vi "Capture@Config__Parameter.vi"(1 "ParamterIn":string) -> (0 "ParamterOut":string)   [LabVIEW 2019]
panel:
  in  "Param":string(combo)
  in  "Config":string(combo)
  in  "CamName":string(combo)
  in  "Confirm":bool
  # "Capture@AddCAM $Capture,$Paramter,$Value"
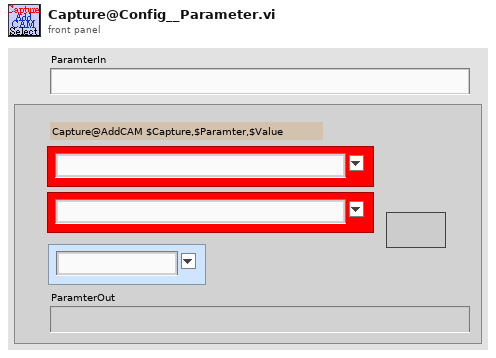
[diagram p1: front panel]
types:
  T1 = enum16{"AddCam", "GetIndex", "Init", "GetList", "SetInfo"}
  T2 = cluster{"Init?":bool, "DeviceName":string, "DeviceInfo":variant, "error state":errorcluster, "Stop":bool}
  T3 = cluster{"Init":refnum<vi>, "Close":refnum<vi>, "Config":refnum<vi>, "NOP":refnum<vi>, "Snapshot":refnum<vi>, "Trigger":refnum<vi>, "GetConfig":refnum<vi>}
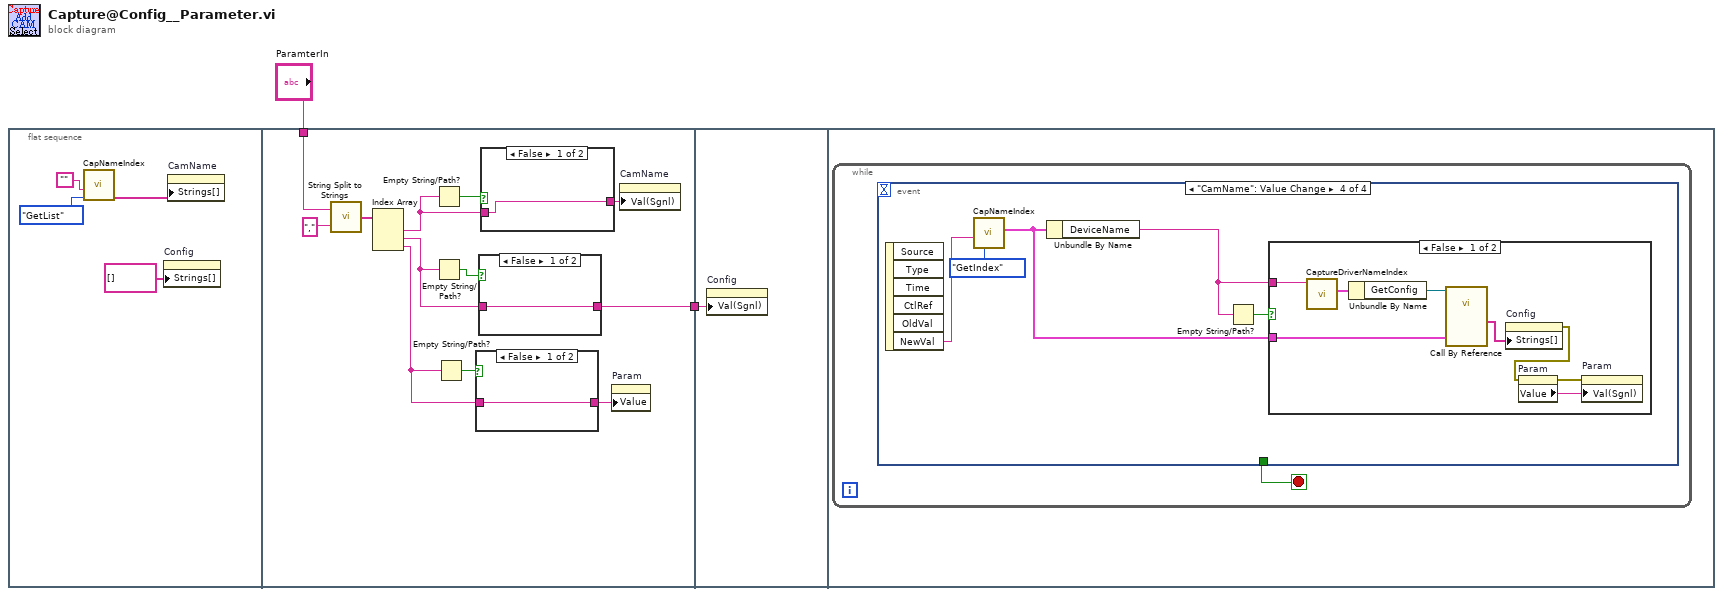
[diagram p0: block diagram]
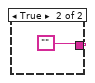
[diagram p2: hidden frame]
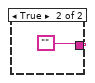
[diagram p3: hidden frame]
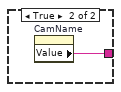
[diagram p4: hidden frame]
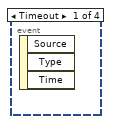
[diagram p5: hidden frame]
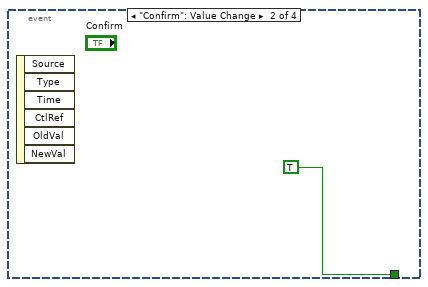
[diagram p6: hidden frame]
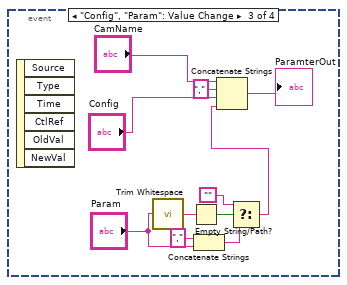
[diagram p7: hidden frame]
diagram:
  n1 = flat-sequence {
    tunnel: "ParamterIn" -> [w16]
    tunnel: [w8] -> w1
    tunnel: w1 -> [w25]
    frame #0 {
      n2 = call "CapNameIndex.vi"("OP"=enum16{"AddCam", "GetIndex", "Init", "GetList"}."GetList", "CamName"="") -> ("DeviceList"=w5:string[])  [unwired: 2 in, 3 out]
      n3 = property on="Config" class="CmbBox"("Strings[]"=string[] [] ("Strings []")) -> ()  [unwired: 2 in, 2 out]
      n4 = property on="CamName" class="CmbBox"("Strings[]"=w5) -> ()  [unwired: 2 in, 2 out]
    }
    frame #1 {
      n5 = call "String Split to Strings.vi"("search string/char (-)"=",", "String"=w16) -> ("Array"=w18:string[])
      n6 = Index Array(array=w18) -> (element #1=w14:string, element #2=w12:string, element #3=w10:string)  [unwired: 3 in]
      n7 = Empty String/Path?(string/path=w14) -> (empty?=w15:bool)
      n8 = Empty String/Path?(string/path=w12) -> (empty?=w13:bool)
      n9 = Empty String/Path?(string/path=w10) -> (empty?=w11:bool)
      n10 = case shown="False" w11 {
        tunnel: [w19 ""] -> w9
        tunnel: w10 -> [w19 _]
        frame False {
        }
        frame True {
        }
      }
      n11 = case shown="False" w13 {
        tunnel: [w21 ""] -> w8
        tunnel: w12 -> [w21 _]
        frame False {
        }
        frame True {
        }
      }
      n12 = case shown="False" w15 {
        tunnel: w14 -> [w23 _]
        tunnel: [w23 w24] -> w7
        frame False {
        }
        frame True {
          n13 = property on="CamName" class="CmbBox"() -> ("Value"=w24:string)  [unwired: 2 in, 2 out]
        }
      }
      n14 = property on="Param" class="CmbBox"("Value"=w9) -> ()  [unwired: 2 in, 2 out]
      n15 = property on="CamName" class="CmbBox"("Val(Sgnl)"=w7) -> ()  [unwired: 2 in, 2 out]
    }
    frame #2 {
      n16 = property on="Config" class="CmbBox"("Val(Sgnl)"=w25) -> ()  [unwired: 2 in, 2 out]
    }
    frame #3 {
      n17 = while {
        stop <- w26 stop-if-true
        n18 = event shown="[3] \"CamName\": Value Change" {
          selector: _ -> [_ _ _ _]
          dyn-events: _ -> [_ _ _ _]
          timeout: _ -> [_ _ _ _]
          tunnel: [_ TRUE _ _] -> w26
          event Timeout {
            n19 = event-data() -> ()  [unwired: 1 in, 3 out]
          }
          event "Confirm": Value Change {
            n20 = event-data() -> ()  [unwired: 1 in, 6 out]
          }
          event "Config", "Param": Value Change {
            n21 = event-data() -> ()  [unwired: 1 in, 6 out]
            n22 = call <vilib>:"Trim Whitespace.vi"("string"="Param") -> ("trimmed string"=w32:string)  [unwired: 1 in]
            n23 = Empty String/Path?(string/path=w32) -> (empty?=w33:bool)
            n24 = Concatenate Strings("," ("string"), "Param") -> (w35:string)
            n25 = Select(t="", s=w33, f=w35) -> (s? t:f=w29:string)
            n26 = Concatenate Strings("CamName", "," ("string"), "Config", w29) -> (→"ParamterOut":string)
          }
          event "CamName": Value Change {
            n27 = event-data() -> ("NewVal"=w43:string)  [unwired: 1 in, 5 out]
            n28 = call "CapNameIndex.vi"("OP"=T1."GetIndex", "CamName"=w43) -> ("DataOut"=w39:T2)  [unwired: 2 in, 3 out]
            n29 = Unbundle By Name(w39) -> ("DeviceName"=w40:string)
            n30 = Empty String/Path?(string/path=w40) -> (empty?=w42:bool)
            n31 = case shown="False" w42 {
              tunnel: w40 -> [w46 _]
              tunnel: w39 -> [w44 _]
              frame False {
                n32 = call "CaptureDriverNameIndex.vi"("Driver"=w46) -> ("DriverVIRef"=w47:T3)  [unwired: 8 in, 2 out]
                n33 = Unbundle By Name(w47) -> ("GetConfig"=w48:refnum<vi>)
                n34 = call-by-ref "?"(reference=w48, "Data in"=w44) -> ("ConfigList"=w45:string[])  [unwired: 4 in, 5 out]
                n35 = property on="Config" class="CmbBox"("Strings[]"=w45) -> (error out=w51:errorcluster)  [unwired: 2 in, 1 out]
                n36 = property on="Param" class="CmbBox"(error in=w51) -> (error out=w50:errorcluster, "Value"=w49:string)  [unwired: 1 in, 1 out]
                n37 = property on="Param" class="CmbBox"(error in=w50, "Val(Sgnl)"=w49) -> ()  [unwired: 1 in, 2 out]
              }
              frame True {
              }
            }
          }
        }
      }
    }
  }
